vi "Handle Error.vi"(8 "error in (no error)":errorcluster, 11 "Server Controller in":refnum<class "Server Controller.lvclass">) -> (0 "error out":errorcluster, 2 "stop actor?":bool=TRUE, 3 "Server Controller out":refnum<class "Server Controller.lvclass">)   [LabVIEW 2026, in "Server Controller.lvlib" / "Server Controller.lvclass"]
doc: "(<B>Filename</B>: Actor Framework.lvlib:Actor.lvclass:Handle Error.vi)\n\nDefines how the actor handles an error that occurred while processing a message.\n\nBy default, this method does nothing except stop the actor. This method also treats error code 43 (coming from <B>error in</B>) as a sign that the actor shut down normally. In this situation, the Handle Error method does not return the error on <B>error out</B>, meaning the actor's caller will not receive it. All other error codes will be returned on <B>error out</B>.\n\nA descendant class may override this method to change this behavior."
uses:
  Server Controller.lvclass
  C:/Program Files/National Instruments/LabVIEW 2026/vi.lib/ActorFramework/Actor/Actor.lvclass
  <vilib>/ActorFramework/Actor/Actor.lvclass/Actor.ctl
  <vilib>/ActorFramework/Message Enqueuer/Message Enqueuer.lvclass/Message Enqueuer.ctl
  <vilib>/ActorFramework/Message Enqueuer/Init from Existing Queue.vi
  recovery/packages/oglib_error-4.2.0.23-323D29123E/File Group 0/user.lib/_OpenG.lib/error/error.llb/Filter Error Codes (Array)__ogtk.vi
  framework/Controller/Controller.lvclass
  <vilib>/ActorFramework/Message Enqueuer/Message Enqueuer.lvclass
  <vilib>/ActorFramework/Actor/Actor.lvclass
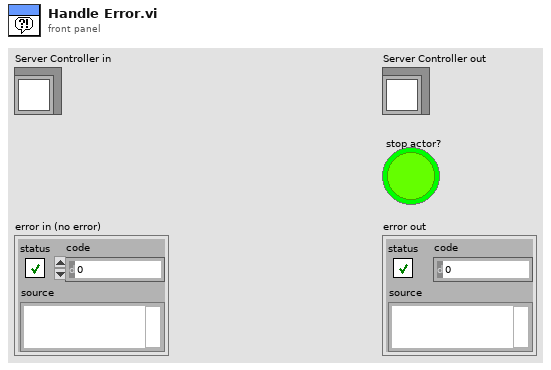
[diagram p1: front panel]
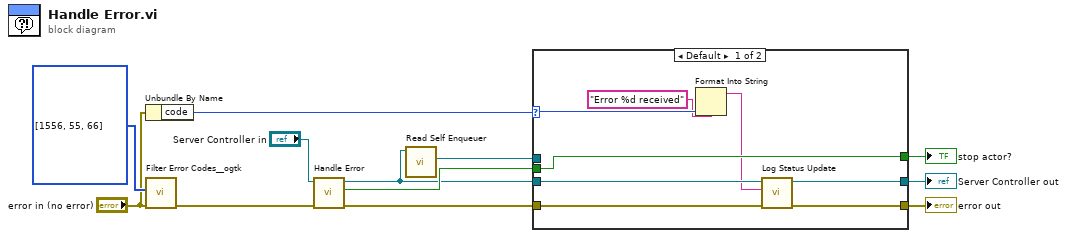
[diagram p0: block diagram]
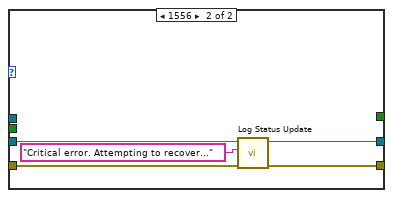
[diagram p2: hidden frame]
diagram:
  n1 = Unbundle By Name("error in (no error)") -> ("code"=w8:i32)
  n2 = call-poly "Filter Error Codes__ogtk.vi"("Error In"="error in (no error)", "Error Codes to Filter"=i32[] [1556, 55, 66]) -> ("Error Out"=w11:errorcluster)  [unwired: 7 in, 2 out]
  n3 = call-parent "Handle Error.vi"("error in (no error)"=w11, "Controller in"="Server Controller in") -> ("error out"=w2:errorcluster, "stop actor?"=w7:bool, "Controller out"=w4:refnum<class "Server Controller.lvclass">)  [unwired: 7 in]
  n4 = call <vilib>:"Read Self Enqueuer.vi"("Actor"=w4) -> ("Self Enqueuer"=w5:refnum<class "Message Enqueuer.lvclass">)  [unwired: 10 in]
  n5 = case shown="Default" w8 {
    selector: w8 -> [w15 _]
    tunnel: [w20 _] -> w6
    tunnel: w7 -> [w20 _]
    tunnel: w5 -> [_ _]
    tunnel: w4 -> [w19 w24]
    tunnel: [w16 w23] -> w3
    tunnel: w2 -> [w18 w22]
    tunnel: [w17 w21] -> w1
    frame Default {
      n6 = Format Into String(format string="Error %d received" ("String"), w15) -> (resulting string=w14:string)  [unwired: 2 in, 1 out]
      n7 = call-dynamic "Log Status Update.vi"("error in (no error)"=w18, "String"=w14, "Controller in"=w19) -> ("error out"=w17:errorcluster, "Controller out"=w16:refnum<class "Server Controller.lvclass">)  [unwired: 7 in]
    }
    frame 1556 {
      n8 = call-dynamic "Log Status Update.vi"("error in (no error)"=w22, "String"="Critical error. Attempting to recover...", "Controller in"=w24) -> ("error out"=w21:errorcluster, "Controller out"=w23:refnum<class "Server Controller.lvclass">)  [unwired: 7 in]
    }
  }
  "Server Controller out" <- w3
  "error out" <- w1
  "stop actor?" <- w6
